vi "Resample (constant to constant,multi-channel).vi"(5 "anti-aliasing?":bool=TRUE, 6 "FIR filter specifications":T1={"alias rejection (dB)"=120.0, "normalized bandwidth"=0.4536} {"normalized bandwidth" format="%.4f"; "alias rejection (dB)" format="%.2f"}, 7 "reset?":bool, 8 "error in (no error)":errorcluster, 9 "dt":dbl=1.0, 10 "delay":dbl, 11 "X":dbl[][](array[numeric]) format="%#.6g") -> (0 "error out":errorcluster, 2 "t0":dbl, 3 "Y":dbl[][](array[numeric]) format="%#.6g")   [LabVIEW 2010, in "NI_AALPro.lvlib"]
doc: "Resamples input signal <B>X</B> according to <B>delay</B> and <B>dt</B> using an FIR filter implementation. Wire data to the <B>X</B> input to determine the polymorphic instance to use or manually select the instance."
uses:
  NI_AALPro.lvlib
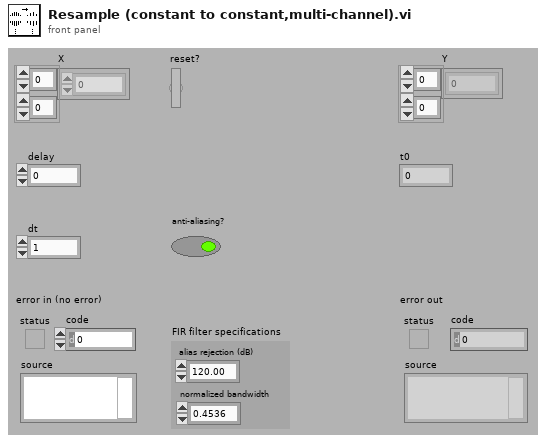
[diagram p1: front panel]
types:
  T1 = cluster{"alias rejection (dB)":dbl, "normalized bandwidth":dbl}
  T2 = cluster{"new sample period":dbl, "Timing Jitter":enum32{"Interpolation", "Rounding"}, "first point location":dbl, "prototype filter":cluster{"h":dbl[], "Max Decimation":i32}}
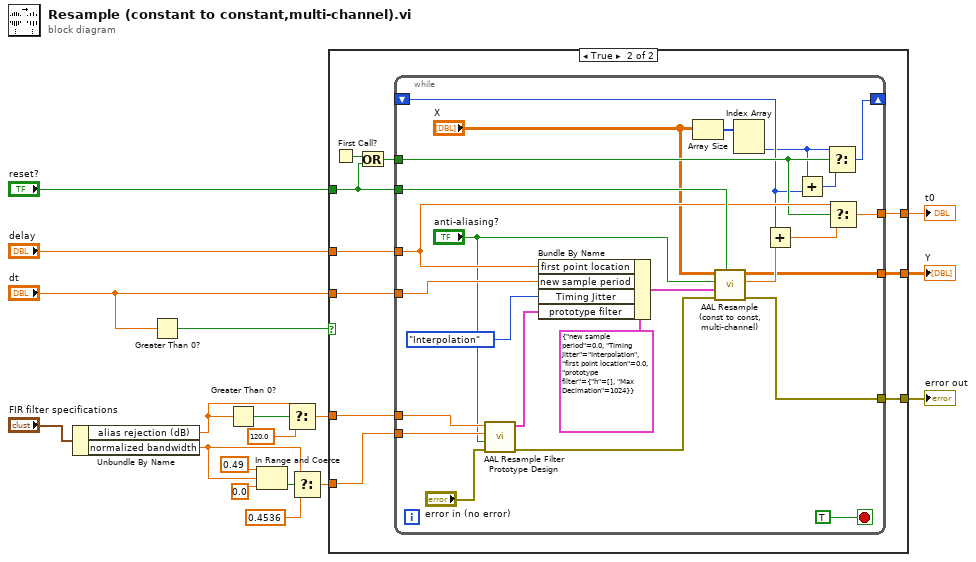
[diagram p0: block diagram]
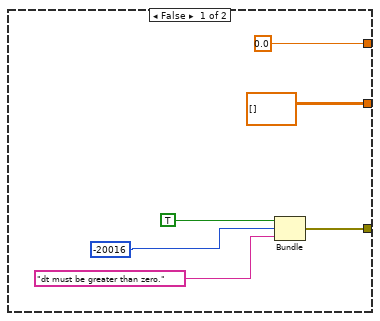
[diagram p2: hidden frame]
diagram:
  n1 = Unbundle By Name("FIR filter specifications") -> ("alias rejection (dB)"=w2:dbl, "normalized bandwidth"=w5:dbl)
  n2 = Greater Than 0?(x="dt") -> (x > 0?=w13:bool)
  n3 = Greater Than 0?(x=w2) -> (x > 0?=w1:bool)
  n4 = In Range and Coerce(upper limit=0.49, x=w5, lower limit=0.0 ("upper limit")) -> (In Range?=w7:bool)  [unwired: 1 out]
  n5 = Select(t=w2, s=w1, f=120.0) -> (s? t:f=w4:dbl)
  n6 = Select(t=w5, s=w7, f=0.4536 ("upper limit")) -> (s? t:f=w3:dbl)
  n7 = case shown="True" w13 {
    tunnel: "dt" -> [_ w32]
    tunnel: "reset?" -> [_ w31]
    tunnel: "delay" -> [_ w30]
    tunnel: [0.0 ("delay") w29] -> w16
    tunnel: [dbl[][] [] ("Y") w28] -> w15
    tunnel: [w22 w27] -> w14
    tunnel: w4 -> [_ w26]
    tunnel: w3 -> [_ w25]
    frame False {
      n8 = Bundle(TRUE, "DtGTZeroErr"=-20016, "dt must be greater than zero.") -> (w22:cluster{bool, "DtGTZeroErr":i32, string})  [unwired: 1 in]
    }
    frame True {
      n9 = First Call?() -> (First Call?: T/F=w34:bool)
      n10 = Or(x=w34, y=w31) -> (x .or. y?=w33:bool)
      n11 = while {
        tunnel: w31 -> [w58]
        tunnel: w30 -> [w49]
        tunnel: w33 -> [w47]
        tunnel: [w51] -> w27
        tunnel: [w48] -> w28
        shift-right: [w44] -> _
        shift-left: _ -> [w41]
        tunnel: [w42] -> w29
        tunnel: w32 -> [w38]
        tunnel: w26 -> [w37]
        tunnel: w25 -> [w36]
        stop <- TRUE stop-if-true
        n12 = call "AAL Resample Filter Prototype Design.vi"("error in (no error)"="error in (no error)", "alias free"="anti-aliasing?", "normalized bandwidth"=w36, "A stop [dB]"=w37) -> ("error out"=w54:errorcluster, "filter prototype"=w55:cluster{"coefficients":dbl[], "factor":i32})  [unwired: 5 in, 1 out]
        n13 = Bundle By Name(cluster=T2 {"new sample period"=0.0, "Timing Jitter"=enum."Interpolation", "first point location"=0.0, "prototype filter"={"h"=[], "Max Decimation"=1024}} ("config"), "first point location"=w49, "new sample period"=w38, "Timing Jitter"=enum32{"Interpolation", "Rounding"}."Interpolation", "prototype filter"=w55) -> (w53:T2)
        n14 = Array Size(array="X") -> (size(s)=w45:i32[])
        n15 = call "AAL Resample (const to const, multi-channel).vi"("reset?"=w58, "error in (no error)"=w54, "config"=w53, "anti-aliasing?"="anti-aliasing?", "X"="X") -> ("error out"=w51:errorcluster, "normalized t0"=w50:dbl, "Y"=w48:dbl[][])  [unwired: 4 in]
        n16 = Index Array(array=w45) -> (element #2=w39:i32)  [unwired: 2 in, 1 out]
        n17 = Add(x=w41, y=w50) -> (x+y=w43:dbl)
        n18 = Add(x=w39, y=w41) -> (x+y=w40:i32)
        n19 = Select(t=w39, s=w47, f=w40) -> (s? t:f=w44:i32)
        n20 = Select(t=w49, s=w47, f=w43) -> (s? t:f=w42:dbl)
      }
    }
  }
  "t0" <- w16
  "error out" <- w14
  "Y" <- w15
